vi "Send status.vi"(8 "error in (no error)":errorcluster, 11 "Channel in":refnum<class "ECHARPE_Channel.lvclass">) -> (0 "error out":errorcluster, 3 "Channel out":refnum<class "ECHARPE_Channel.lvclass">)   [LabVIEW 2018, in "ECHARPE_Channel.lvclass"]
uses:
  ECHARPE_Channel.lvclass
  C:/Users/Denis/Desktop/S4ACS/S4ACS/Channel/Channel.lvclass
  Server/Server.lvclass/Server.ctl
  Sim_CCD/Sim_CCD.lvclass/Sim_CCD.ctl
  RxTx/RxTx.lvclass
  Sim_CCD/Sim_CCD.lvclass
  Server/Server.lvclass
  Channel/Channel.lvclass
panel:
  in  "status message":T1
  in  "Camera Status":T2
  in  "comm status":T3
  in  "Prev SET parameters":T4
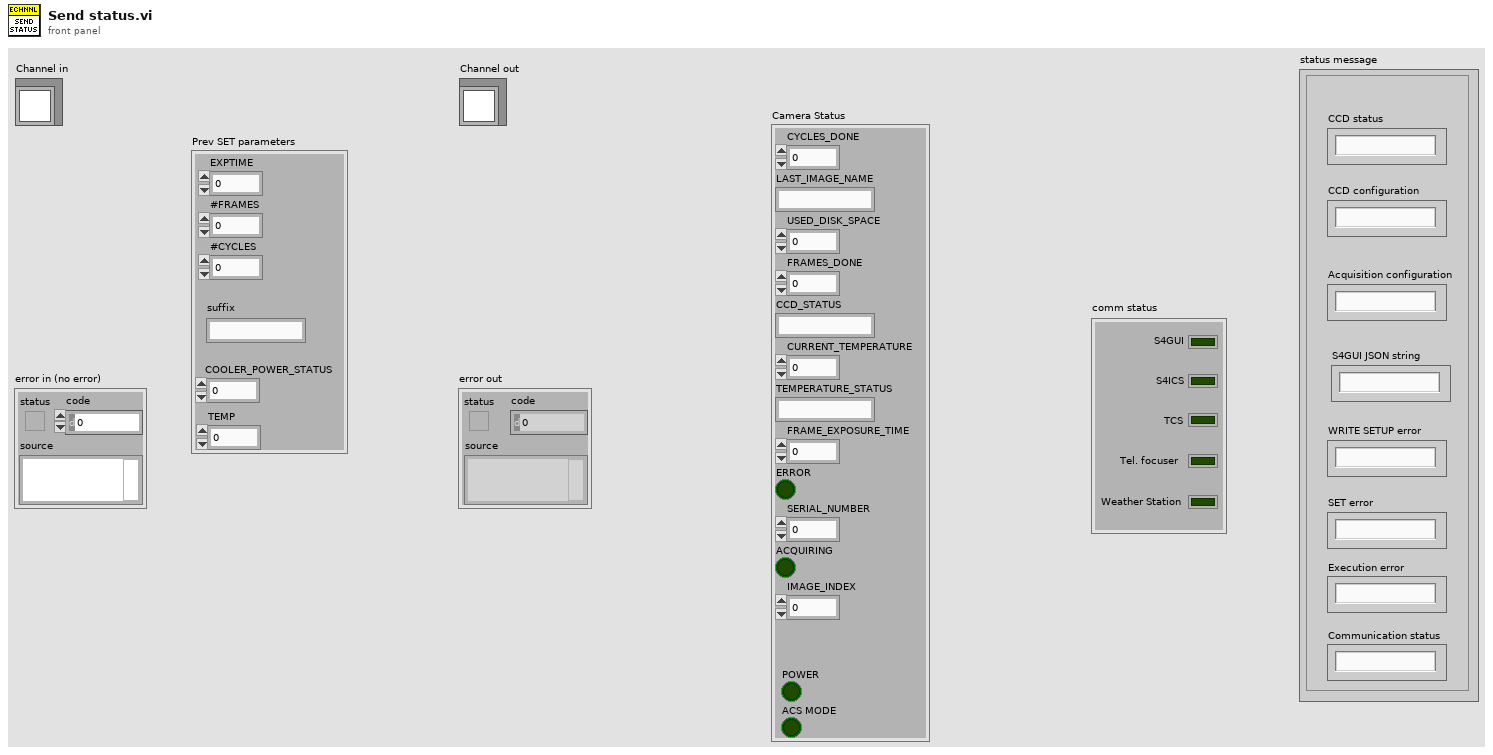
[diagram p1: front panel]
types:
  T1 = cluster{"CCD status":string, "CCD configuration":string, "Acquisition configuration":string, "S4GUI JSON string":string, "WRITE SETUP error":string, "Execution error":string, "SET error":string, "Communication status":string}
  T2 = cluster{"CYCLES_DONE":u16, "LAST_IMAGE_NAME":string, "USED_DISK_SPACE":u16, "FRAMES_DONE":u16, "CCD_STATUS":string, "CURRENT_TEMPERATURE":i16, "TEMPERATURE_STATUS":string, "FRAME_EXPOSURE_TIME":sgl, "ERROR":bool, "SERIAL_NUMBER":u16, "ACQUIRING":bool, "IMAGE_INDEX":u32, "POWER":bool, "ACS MODE":bool}
  T3 = cluster{"S4GUI":bool, "S4ICS":bool, "TCS":bool, "Weather Station":bool, "Tel. focuser":bool}
  T4 = cluster{"EXPTIME":dbl, "#FRAMES":u32, "#CYCLES":u32, "suffix":string, "COOLER_POWER_STATUS":u8, "TEMP":i32}
  T5 = cluster{"CYCLES_DONE":u16, "LAST_IMAGE_NAME":string, "USED_DISK_SPACE":u16, "IMAGE_INDEX":u32, "acquisition error":bool}
  T6 = cluster{"State Machine.lvclass":refnum<class "State Machine.lvclass">, "RxTx.lvclass":refnum<class "RxTx.lvclass">, "Save_Header_RxTx.lvclass":refnum<class "RxTx.lvclass">, "Status SM.lvclass":refnum<class "State Machine.lvclass">, "Status RxTx.lvclass":refnum<class "RxTx.lvclass">, "servers array":refnum<class "Server.lvclass">[], "Events log file.lvclass":refnum<class "Log File.lvclass">, "Errors log file.lvclass":refnum<class "Log File.lvclass">, "Keywords log file.lvclass":refnum<class "Log File.lvclass">, "Sim_CCD.lvclass":refnum<class "Sim_CCD.lvclass">}
  T7 = cluster{"FRAMES_DONE":u16, "CCD_STATUS":string, "CURRENT_TEMPERATURE":i16, "TEMPERATURE_STATUS":string, "FRAME_EXPOSURE_TIME":dbl, "SERIAL_NUMBER":u16, "ACQUIRING":bool, "POWER":bool, "ACS MODE":bool}
  T8 = cluster{"PREAMP":u16, "READOUT_RATE":u16, "VERTICAL_SHIFT_SPEED":u16, "READ_MODE":u16, "VERTICAL_CLOCK_VOLTAGE":u16, "ACQUISITION_MODE":u16, "AD_CHANNEL":u16, "SHUTTER_TTL":u16, "SHUTTER_OPENING_TIME":u16, "SHUTTER_CLOSING_TIME":u16, "SHUTTER_MODE":u16, "TRIGGER_MODE":u16, "VBIN":u16, "INITIAL_LINE":u16, "INITIAL_COLUMN":u16, "FINAL_LINE":u16, "FINAL_COLUMN":u16, "HBIN":u16}
  T9 = cluster{"EXPTIME":dbl, "#FRAMES":u32, "COOLER_POWER_STATUS":u16, "TEMP":i32}
  T10 = cluster{"EXPTIME":errorcluster, "#FRAMES":errorcluster, "COOLER_POWER_STATUS":errorcluster, "TEMP":errorcluster}
  T11 = cluster{"CCD status":string, "camera op mode":string, "acq config":string, "GUI status msg":string, "op mode errors":string, "acq config error":string, "comm status":string}
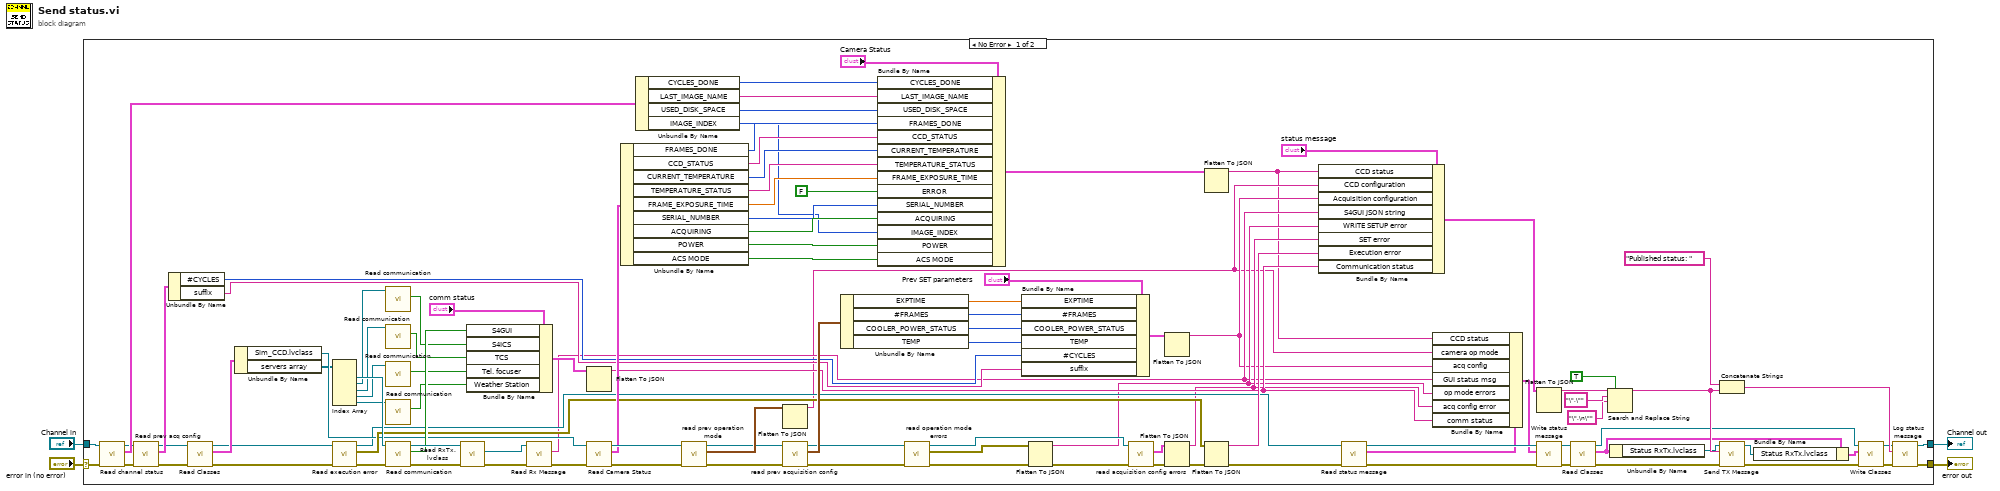
[diagram p0: block diagram]
diagram:
  n1 = case shown="No Error" "error in (no error)" {
    selector: "error in (no error)" -> [w36 w114]
    tunnel: [w68 w114] -> w3
    tunnel: [w67 w113] -> w1
    tunnel: "Channel in" -> [w35 w113]
    frame No Error {
      n2 = call-dynamic "Read channel status.vi"("error in (no error)"=w36, "Channel in"=w35) -> ("error out"=w38:errorcluster, "channel status"=w48:T5, "Channel out"=w37:refnum<class "ECHARPE_Channel.lvclass">)  [unwired: 7 in]
      n3 = call-dynamic "Read prev acq config.vi"("error in (no error)"=w38, "Channel in"=w37) -> ("error out"=w40:errorcluster, "prev acq config"=w47:cluster{"suffix":string, "#CYCLES":u32}, "Channel out"=w39:refnum<class "ECHARPE_Channel.lvclass">)  [unwired: 7 in]
      n4 = Unbundle By Name(w47) -> ("#CYCLES"=w45:u32, "suffix"=w46:string)
      n5 = call-dynamic "Read Classes.vi"("error in (no error)"=w40, "Channel in"=w39) -> ("error out"=w33:errorcluster, "Classes"=w43:T6, "Channel out"=w34:refnum<class "ECHARPE_Channel.lvclass">)  [unwired: 7 in]
      n6 = Unbundle By Name(w43) -> ("Sim_CCD.lvclass"=w42:refnum<class "Sim_CCD.lvclass">, "servers array"=w41:refnum<class "Server.lvclass">[])
      n7 = Index Array(array=w41) -> (element #1=w82:refnum<class "Server.lvclass">, element #2=w79:refnum<class "Server.lvclass">, element #3=w78:refnum<class "Server.lvclass">, element #4=w77:refnum<class "Server.lvclass">, element #5=w76:refnum<class "Server.lvclass">)  [unwired: 5 in]
      n8 = call-dynamic "Read execution error.vi"("error in (no error)"=w33, "Channel in"=w34) -> ("error out"=w32:errorcluster, "execution error"=w44:errorcluster, "Channel out"=w31:refnum<class "ECHARPE_Channel.lvclass">)  [unwired: 7 in]
      n9 = call "Read communication.vi"("Server in"=w79) -> ("communication"=w73:bool)  [unwired: 8 in, 2 out]
      n10 = call "Read communication.vi"("Server in"=w78) -> ("communication"=w72:bool)  [unwired: 8 in, 2 out]
      n11 = call "Read communication.vi"("Server in"=w77) -> ("communication"=w71:bool)  [unwired: 8 in, 2 out]
      n12 = call "Read communication.vi"("Server in"=w76) -> ("communication"=w70:bool)  [unwired: 8 in, 2 out]
      n13 = call "Read communication.vi"("error in (no error)"=w32, "Server in"=w82) -> ("error out"=w80:errorcluster, "communication"=w74:bool, "Server out"=w81:refnum<class "Server.lvclass">)  [unwired: 7 in]
      n14 = call "Read RxTx.lvclass.vi"("error in (no error)"=w80, "Server in"=w81) -> ("error out"=w97:errorcluster, "RxTx.lvclass"=w98:refnum<class "RxTx.lvclass">)  [unwired: 7 in, 1 out]
      n15 = Bundle By Name(cluster="comm status", "S4GUI"=w74, "S4ICS"=w73, "TCS"=w72, "Tel. focuser"=w71, "Weather Station"=w70) -> (w69:T3)
      n16 = call "Read Rx Message.vi"("error in (no error)"=w97, "RxTx in"=w98) -> ("error out"=w96:errorcluster, "Rx Message"=w12:string)  [unwired: 7 in, 1 out]
      n17 = Flatten To JSON(anything=w69) -> (JSON string=w15:string)  [unwired: 2 in, 1 out]
      n18 = call "Read Camera Status.vi"("error in (no error)"=w96, "CCDCamera in"=w42) -> ("error out"=w110:errorcluster, "camera status"=w61:T7, "CCDCamera out"=w111:refnum<class "Sim_CCD.lvclass">)  [unwired: 7 in]
      n19 = Unbundle By Name(w61) -> ("FRAMES_DONE"=w54:u16, "CCD_STATUS"=w55:string, "CURRENT_TEMPERATURE"=w56:i16, "TEMPERATURE_STATUS"=w57:string, "FRAME_EXPOSURE_TIME"=w58:dbl, "SERIAL_NUMBER"=w59:u16, "ACQUIRING"=w60:bool, "POWER"=w8:bool, "ACS MODE"=w7:bool)
      n20 = Unbundle By Name(w48) -> ("CYCLES_DONE"=w53:u16, "LAST_IMAGE_NAME"=w52:string, "USED_DISK_SPACE"=w51:u16, "IMAGE_INDEX"=w50:u32)
      n21 = call "read prev operation mode.vi"("error in (no error)"=w110, "Simulated_CCD_Camera in"=w111) -> ("error out"=w108:errorcluster, "prev operation mode"=w112:T8, "Simulated_CCD_Camera out"=w109:refnum<class "Sim_CCD.lvclass">)  [unwired: 7 in]
      n22 = Flatten To JSON(anything=w112) -> (JSON string=w10:string)  [unwired: 2 in, 1 out]
      n23 = call "read prev acquisition config.vi"("error in (no error)"=w108, "Simulated_CCD_Camera in"=w109) -> ("error out"=w93:errorcluster, "prev acquisition configuration"=w101:T9, "Simulated_CCD_Camera out"=w91:refnum<class "Sim_CCD.lvclass">)  [unwired: 7 in]
      n24 = Unbundle By Name(w101) -> ("EXPTIME"=w100:dbl, "#FRAMES"=w99:u32, "COOLER_POWER_STATUS"=w5:u16, "TEMP"=w6:i32)
      n25 = Bundle By Name(cluster="Camera Status", "CYCLES_DONE"=w53, "LAST_IMAGE_NAME"=w52, "USED_DISK_SPACE"=w51, "FRAMES_DONE"=w54, "CCD_STATUS"=w55, "CURRENT_TEMPERATURE"=w56, "TEMPERATURE_STATUS"=w57, "FRAME_EXPOSURE_TIME"=w58, "ERROR"=FALSE, "SERIAL_NUMBER"=w59, "ACQUIRING"=w60, "IMAGE_INDEX"=w50, "POWER"=w8, "ACS MODE"=w7) -> (w62:T2)
      n26 = call "read operation mode errors.vi"("error in (no error)"=w93, "Simulated_CCD_Camera in"=w91) -> ("error out"=w86:errorcluster, "WRITE SETUP errors"=w87:errorcluster[], "Simulated_CCD_Camera out"=w92:refnum<class "Sim_CCD.lvclass">)  [unwired: 7 in]
      n27 = Bundle By Name(cluster="Prev SET parameters", "EXPTIME"=w100, "#FRAMES"=w99, "COOLER_POWER_STATUS"=w5, "TEMP"=w6, "#CYCLES"=w45, "suffix"=w46) -> (w102:T4)
      n28 = Flatten To JSON(anything=w87, error in (no error)=w86) -> (JSON string=w13:string, 11:w85:errorcluster)  [unwired: 1 in]
      n29 = call "read acquisition config errors.vi"("error in (no error)"=w85, "Simulated Camera in"=w92) -> ("error out"=w90:errorcluster, "acquisition config errors"=w84:T10)  [unwired: 7 in, 1 out]
      n30 = Flatten To JSON(anything=w102) -> (JSON string=w11:string)  [unwired: 2 in, 1 out]
      n31 = Flatten To JSON(anything=w84, error in (no error)=w90) -> (JSON string=w14:string, 11:w89:errorcluster)  [unwired: 1 in]
      n32 = Flatten To JSON(anything=w62) -> (JSON string=w9:string)  [unwired: 2 in, 1 out]
      n33 = Flatten To JSON(anything=w44, error in (no error)=w89) -> (JSON string=w83:string, 11:w88:errorcluster)  [unwired: 1 in]
      n34 = Bundle By Name(cluster="status message", "CCD status"=w9, "CCD configuration"=w10, "Acquisition configuration"=w11, "S4GUI JSON string"=w12, "WRITE SETUP error"=w13, "SET error"=w14, "Execution error"=w83, "Communication status"=w15) -> (w16:T1)
      n35 = call "Read status message.vi"("error in (no error)"=w88, "Channel in"=w31) -> ("error out"=w94:errorcluster, "status message"=w18:T11, "Channel out"=w95:refnum<class "ECHARPE_Channel.lvclass">)  [unwired: 7 in]
      n36 = Bundle By Name(cluster=w18, "CCD status"=w9, "camera op mode"=w10, "acq config"=w11, "GUI status msg"=w12, "op mode errors"=w13, "acq config error"=w14, "comm status"=w15) -> (w17:T11)
      n37 = Flatten To JSON(anything=w16) -> (JSON string=w107:string)  [unwired: 2 in, 1 out]
      n38 = call "Write status message.vi"("error in (no error)"=w94, "status message"=w17, "Channel in"=w95) -> ("error out"=w28:errorcluster, "Channel out"=w27:refnum<class "ECHARPE_Channel.lvclass">)  [unwired: 7 in]
      n39 = call-dynamic "Read Classes.vi"("error in (no error)"=w28, "Channel in"=w27) -> ("error out"=w25:errorcluster, "Classes"=w24:T6, "Channel out"=w22:refnum<class "ECHARPE_Channel.lvclass">)  [unwired: 7 in]
      n40 = Search and Replace String(replace all?=TRUE ("replace all? (F)"), input string=w107, search string="\",\"", replace string="\",\n\"" ("search string")) -> (result string=w66:string)  [unwired: 4 in, 3 out]
      n41 = Unbundle By Name(w24) -> ("Status RxTx.lvclass"=w26:refnum<class "RxTx.lvclass">)
      n42 = Concatenate Strings("Published status: " ("string"), w66) -> (w65:string)
      n43 = call "Send TX Message.vi"("error in (no error)"=w25, "message"=w66, "RxTx in"=w26) -> ("error out"=w21:errorcluster, "RxTx out"=w20:refnum<class "RxTx.lvclass">)  [unwired: 7 in]
      n44 = Bundle By Name(cluster=w24, "Status RxTx.lvclass"=w20) -> (w23:T6)
      n45 = call-dynamic "Write Classes.vi"("error in (no error)"=w21, "Classes"=w23, "Channel in"=w22) -> ("error out"=w30:errorcluster, "Channel out"=w29:refnum<class "ECHARPE_Channel.lvclass">)  [unwired: 7 in]
      n46 = call "Log status message.vi"("error in (no error)"=w30, "String"=w65, "Channel in"=w29) -> ("error out"=w68:errorcluster, "Channel out"=w67:refnum<class "ECHARPE_Channel.lvclass">)  [unwired: 7 in]
    }
    frame Error {
    }
  }
  "error out" <- w3
  "Channel out" <- w1
